vi "CSMP-Register Status.vi"(0 "state":string, 1 "args":string, 2 "source/target":string, 5 "Error in":errorcluster caption="Error in (no error)", 8 "Module Name":string) -> (14 "state out":string, 15 "args out":string, 16 "source/target out":string, 17 "Pre-State out":string, 18 "Pre-Args out":string, 19 "error":errorcluster)   [LabVIEW 2020, in "Communicable State Machine.lvlib"]
uses:
  Communicable State Machine.lvlib
  CSM - Make String Arguments Safe.vi
  CSM - Keywords.vi
  FGV-BroadcastRegistry.vi
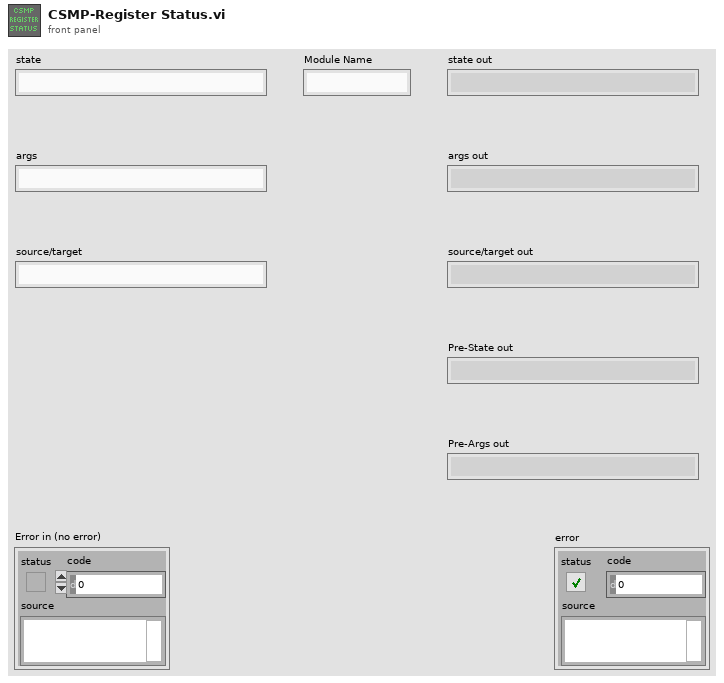
[diagram p1: front panel]
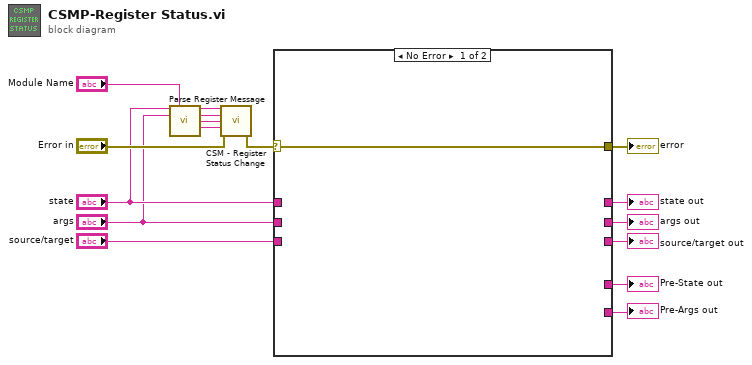
[diagram p0: block diagram]
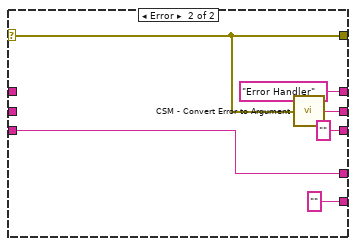
[diagram p2: hidden frame]
diagram:
  n1 = call "Parse Register Message.vi"("state"="state", "Module Name"="Module Name", "args"="args") -> ("target"=w4:string, "source"=w3:string, "status"=w2:string, "api"=w1:string)  [unwired: 9 in]
  n2 = call "CSM - Register Status Change.vi"("CSM Name"=w4, "Source CSM Name (* as Default)"=w3, "Status"=w2, "Response Message (if \"\", same as Source Message)"=w1, "Error in"="Error in") -> ("Error out"=w14:errorcluster)  [unwired: 9 in, 1 out]
  n3 = case shown="No Error" w14 {
    selector: w14 -> [w17 w21]
    tunnel: [_ w19] -> w15
    tunnel: [w17 w21] -> w13
    tunnel: [_ "" ("Pre-State out")] -> w12
    tunnel: "state" -> [_ _]
    tunnel: [_ "Error Handler" ("state")] -> w11
    tunnel: "args" -> [_ _]
    tunnel: [_ w20] -> w10
    tunnel: "source/target" -> [_ w19]
    tunnel: [_ "" ("source/target")] -> w8
    frame No Error {
    }
    frame Error {
      n4 = call "CSM - Convert Error to Argument.vi"("error in (no error)"=w21) -> ("Arguments"=w20:string)  [unwired: 4 in]
    }
  }
  "state out" <- w11
  "args out" <- w10
  "source/target out" <- w8
  "Pre-State out" <- w15
  "Pre-Args out" <- w12
  "error" <- w13
